vi "normalize_by_pixelhits.vi"(8 "error in":errorcluster, 10 "Pixelhits array":refnum<data-value>, 11 "Image in":dbl[][](array[numeric])) -> (0 "error out":errorcluster, 3 "Image out":dbl[][](array[numeric]))   [LabVIEW 2011, in "Fiberscope_library.lvlib"]
uses:
  Fiberscope_library.lvlib
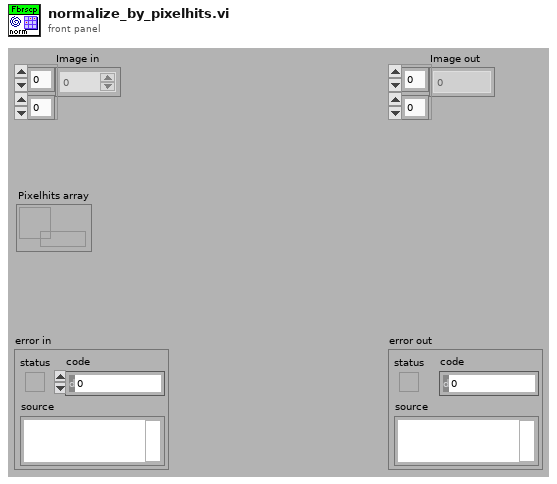
[diagram p1: front panel]
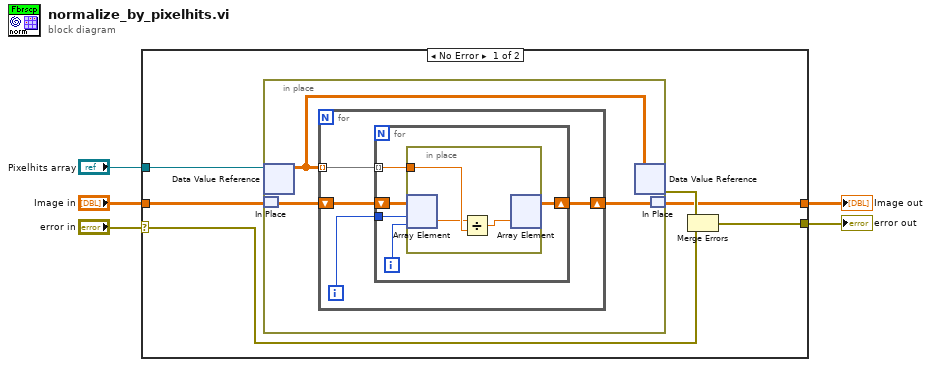
[diagram p0: block diagram]
diagram:
  n1 = case shown="No Error" "error in" {
    selector: "error in" -> [w10 w27]
    tunnel: [w9 w27] -> w4
    tunnel: "Pixelhits array" -> [w11 _]
    tunnel: "Image in" -> [w7 _]
    tunnel: [w6 _] -> w1
    frame No Error {
      n2 = in-place {
        n3 = in-place-dvr #1(w11) -> (w14:dbl[][])  [unwired: 1 out]
        n4 = in-place-match #2(w7) -> (w13:dbl[][])
        n5 = for {
          shift-right: [w15] -> w12
          shift-left: w13 -> [w17]
          tunnel: w14 -> [w18] mode=indexing
          i -> [w16]
          n6 = for {
            tunnel: w18 -> [w21] mode=indexing
            shift-right: [w19] -> w15
            shift-left: w17 -> [w20]
            tunnel: w16 -> [w23]
            i -> [w22]
            n7 = in-place {
              in-place-border: w21 -> [w26]
              n8 = in-place-array #3(w20, w23, w22) -> (w25:dbl)
              n9 = Divide(x=w25, y=w26) -> (x/y=w24:dbl)
              n10 = in-place-array #3(w24) -> (w19:dbl[][])  [unwired: 2 out]
            }
          }
        }
        n11 = in-place-dvr #1(w14) -> (w8:errorcluster)  [unwired: 1 out]
        n12 = in-place-match #2(w12) -> (w6:dbl[][])
      }
      n13 = Merge Errors(w8, w10) -> (w9:errorcluster)
    }
    frame Error {
    }
  }
  "error out" <- w4
  "Image out" <- w1
